vi "Logging Message Loop.vi"(8 "error in (no error)":errorcluster, 10 "Data Queue":refnum<queue>, 11 "Message Queues":T2) -> (0 "error out":errorcluster)   [LabVIEW 2018, in "System Logging.lvlib" / "Logging.lvlib"]
doc: "The message loop subVI to handle messages pertaining to logging data."
uses:
  Logging.lvlib
  Logging Configuration.ctl
  support/Message Queue/Message Queue.lvlib
  Logging State.ctl
  <vilib>/ErrorRing/Error Ring.xnode
  <vilib>/Utility/error.llb/Error Cluster From Error Code.vi
  support/Message Queue/Message Cluster.ctl
  support/Message Queue/All Message Queues.ctl
  Valve Time Stamp.ctl
panel:
  out "Numeric":i32
  out "Boolean 4":bool=TRUE
  out "Boolean 3":bool=TRUE
  out "Boolean 2":bool=TRUE
  out "Trigger times logged":bool=TRUE
  out "Boolean":bool=TRUE
  in  "Cluster 3":T1
  in  "Cluster 2":T1
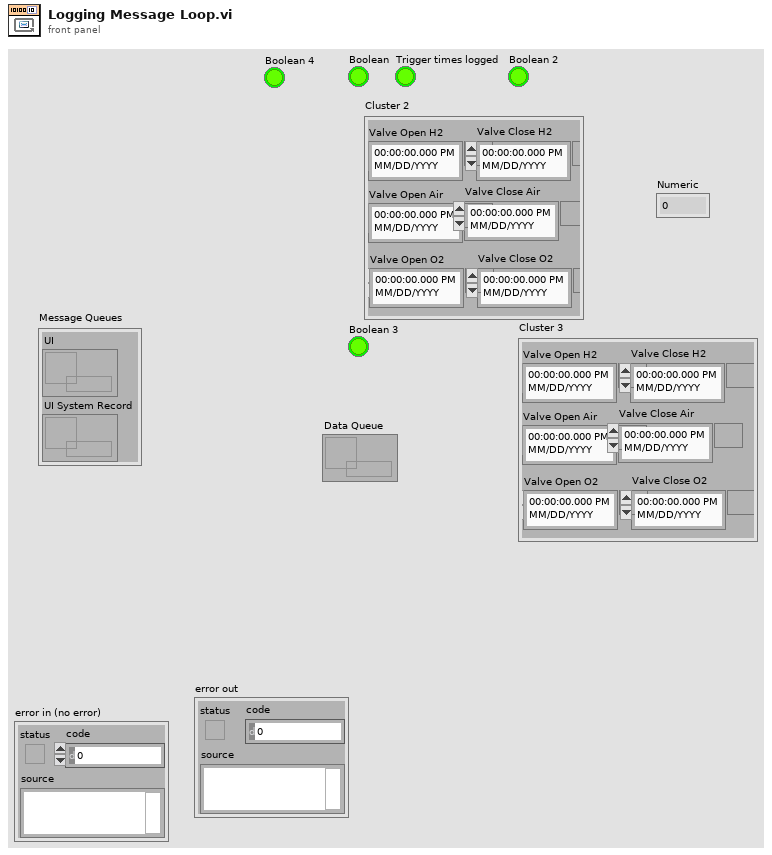
[diagram p1: front panel]
types:
  T1 = typedef "System Logging.lvlib/Valve Time Stamp.ctl" = cluster{"Valve Open Air":timestamp, "Valve Close Air":timestamp, "Valve Open H2":timestamp, "Valve Close H2":timestamp, "Valve Open O2":timestamp, "Valve Close O2":timestamp}
  T2 = typedef "Message Queue.lvlib/All Message Queues.ctl" = cluster{"UI":refnum<queue>, "UI System Record":refnum<queue>}
  T3 = typedef "System Logging.lvlib/Logging.lvlib/Logging State.ctl" = enum16{"Idle", "Logging"}
  T4 = enum16{"open", "open or create", "create or replace", "create", "open (read-only)"}
  T5 = typedef "System Logging.lvlib/Logging.lvlib/Logging Configuration.ctl" = cluster{"Log File Base Path":path, "TDMS File Reference":refnum<k34>, "Log File Base Path 2":path, "TDMS File Reference 2":refnum<k34>}
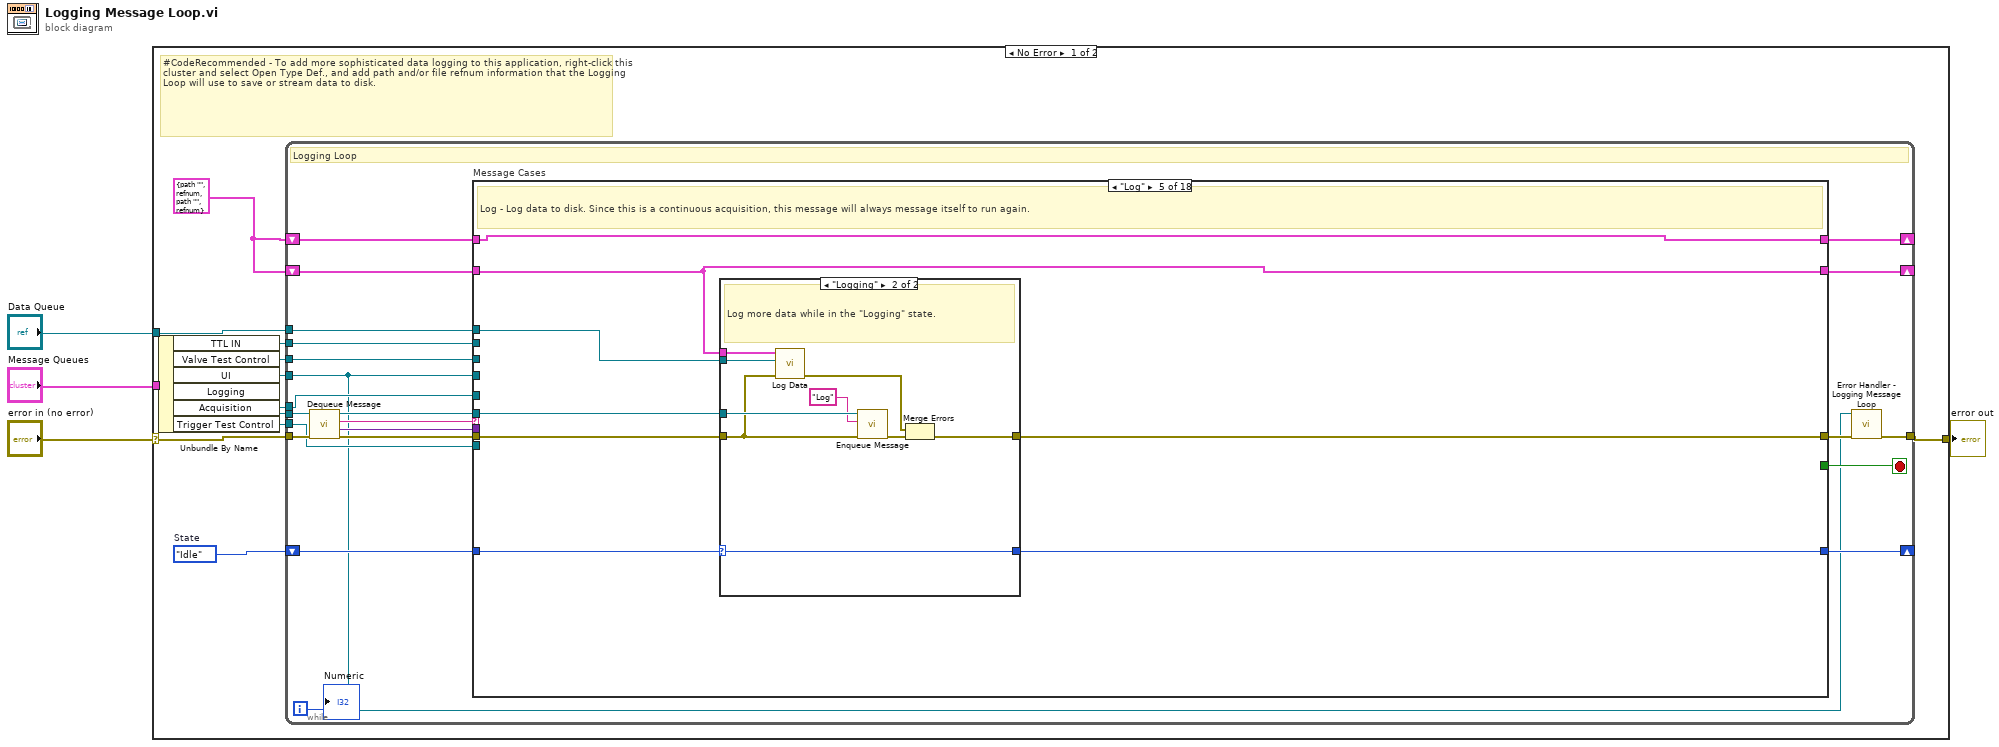
[diagram p0: block diagram]
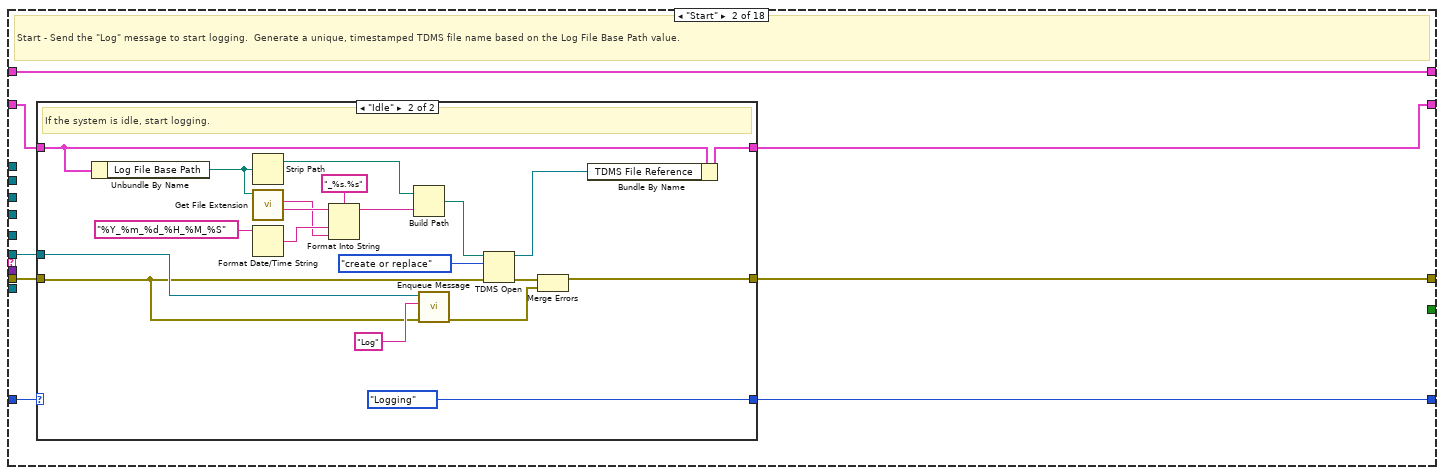
[diagram p3: hidden frame]
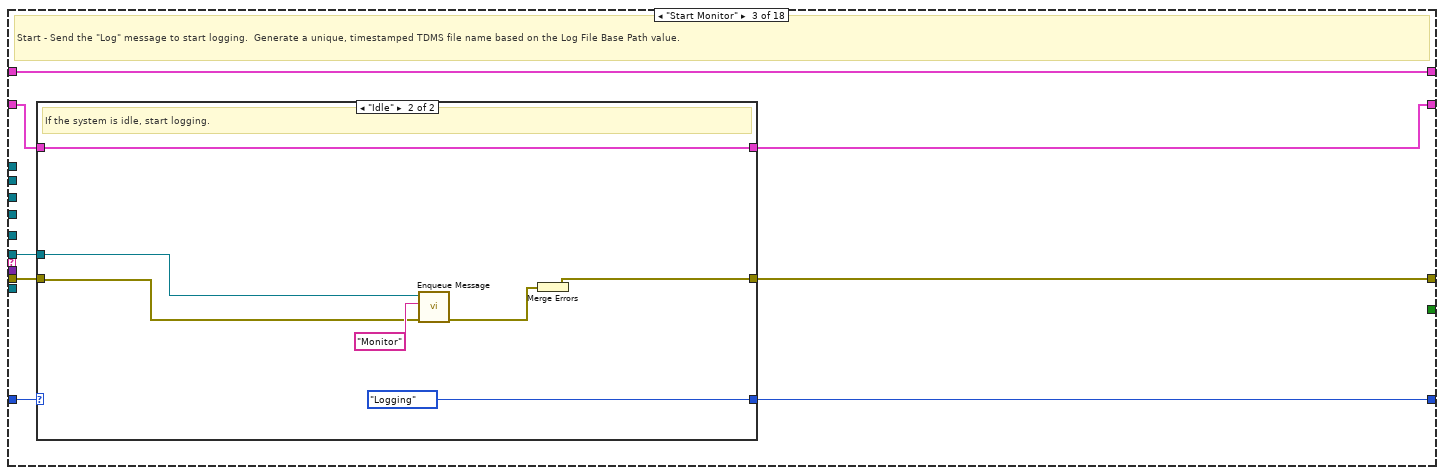
[diagram p5: hidden frame]
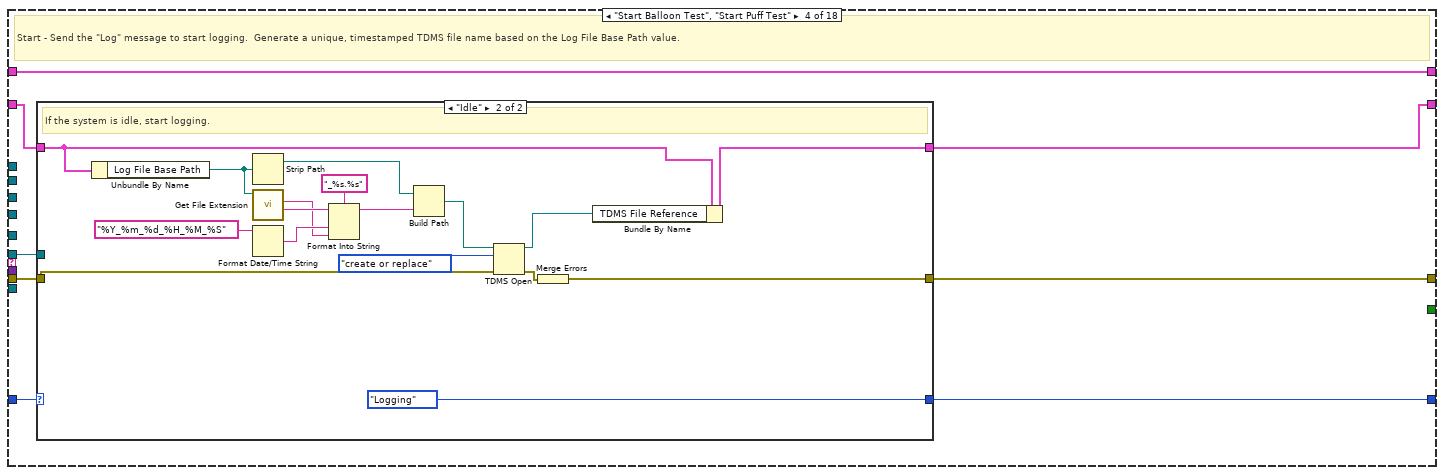
[diagram p7: hidden frame]
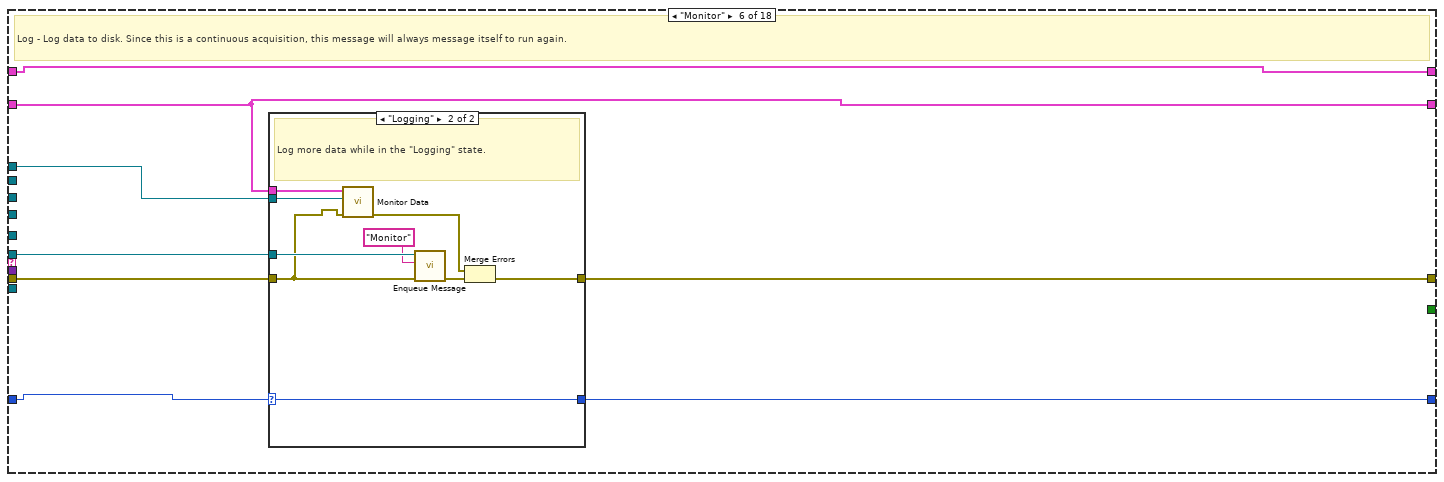
[diagram p10: hidden frame]
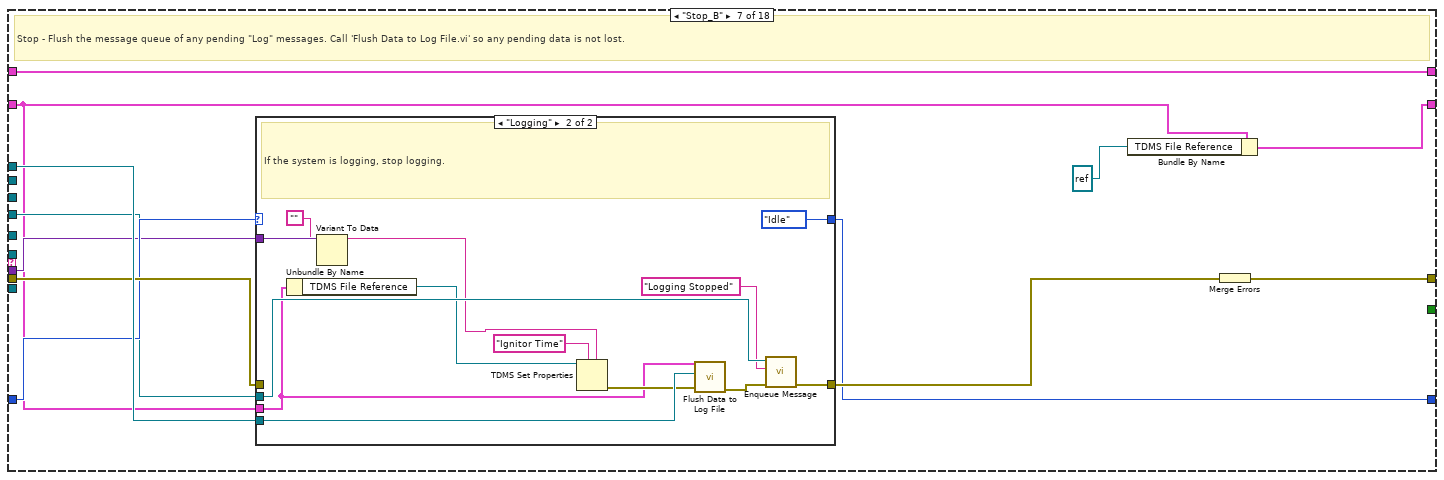
[diagram p12: hidden frame]
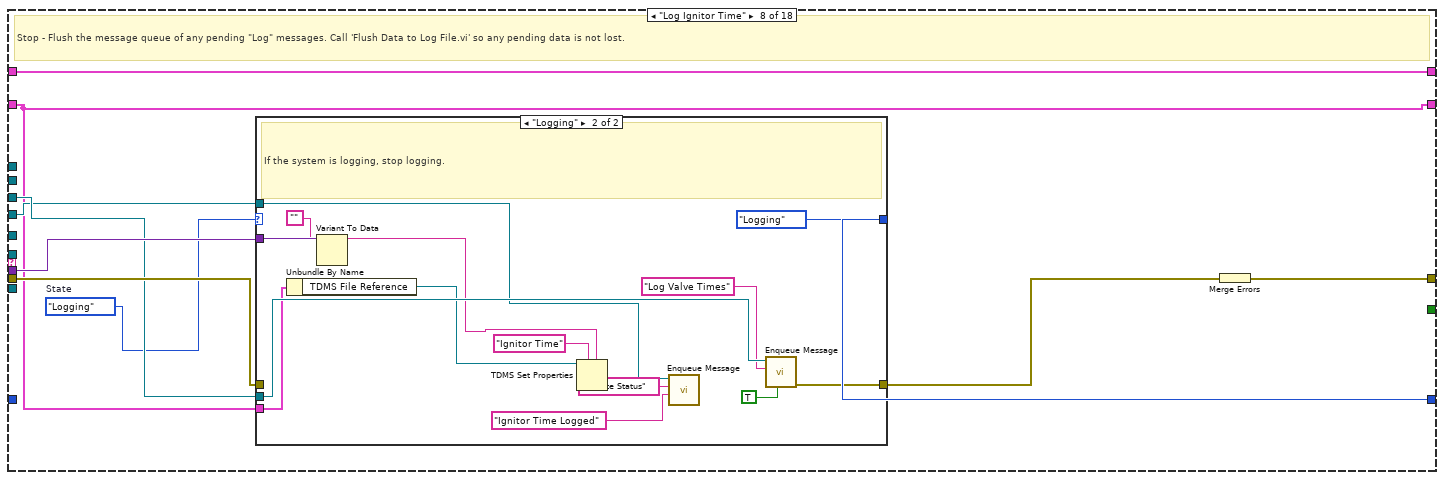
[diagram p14: hidden frame]
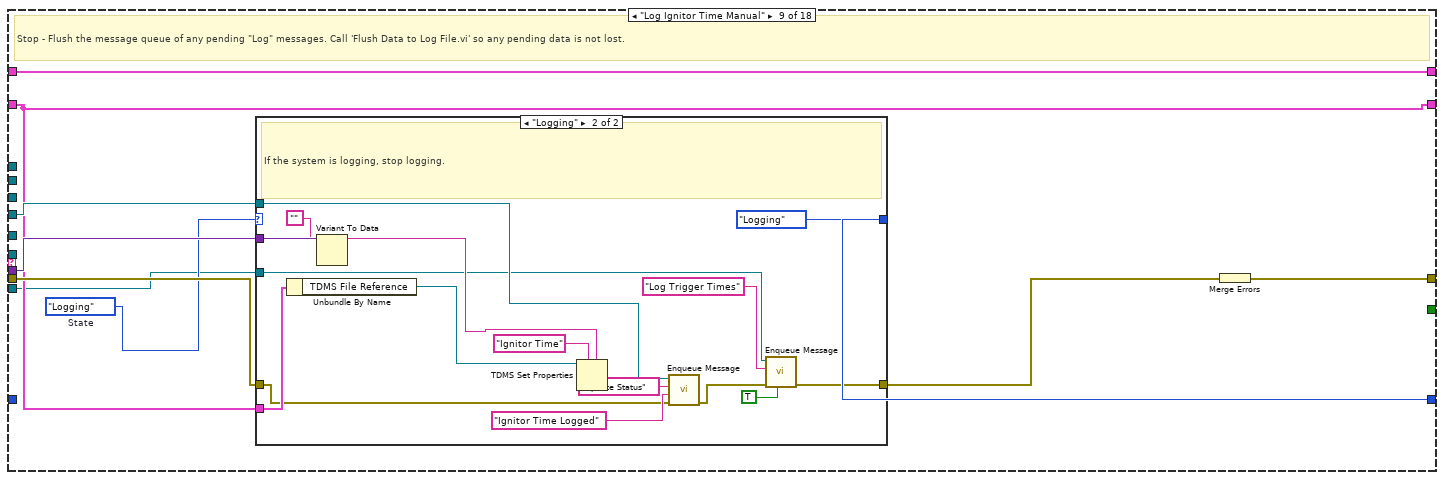
[diagram p16: hidden frame]
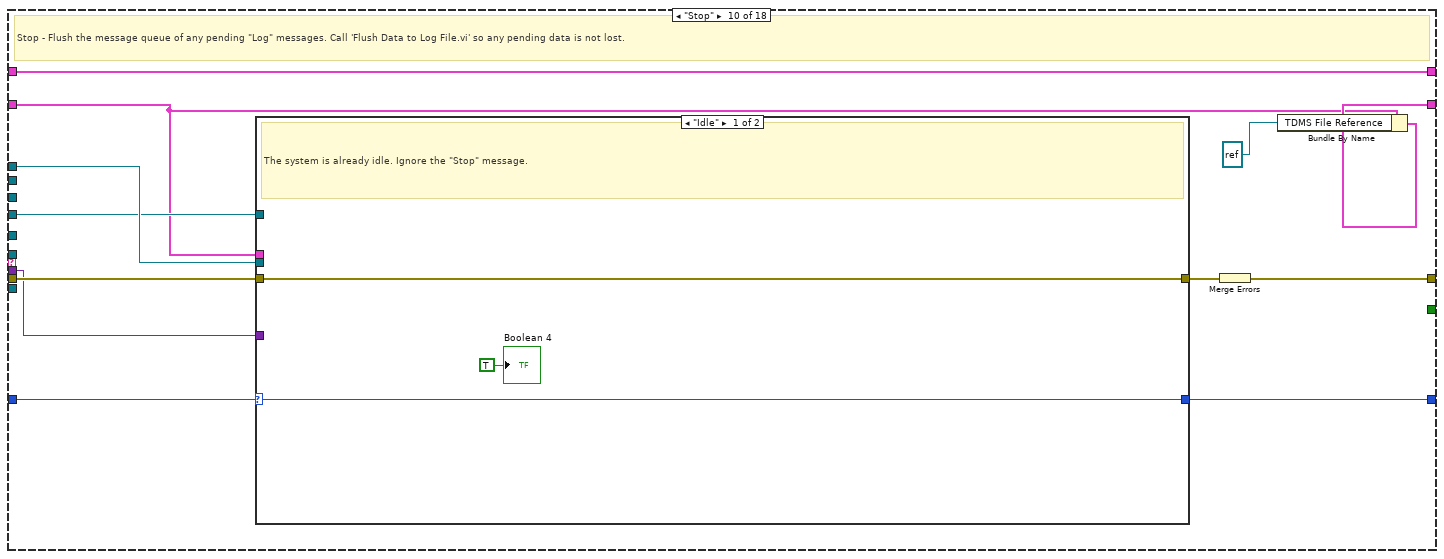
[diagram p18: hidden frame]
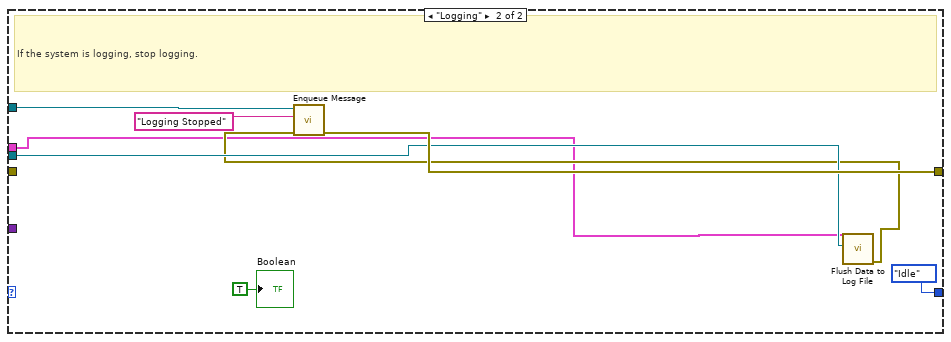
[diagram p19: hidden frame]
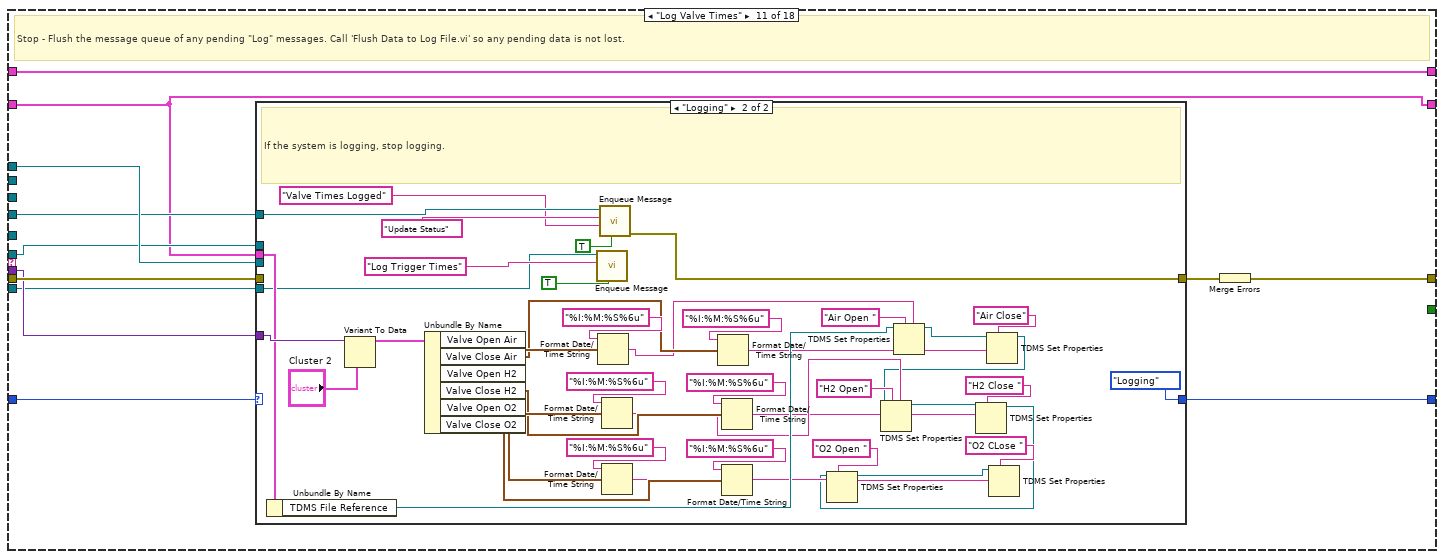
[diagram p20: hidden frame]
diagram:
  n1 = case shown="No Error" "error in (no error)" {
    selector: "error in (no error)" -> [w13 w506]
    tunnel: "Message Queues" -> [w16 _]
    tunnel: [w14 w506] -> w3
    tunnel: "Data Queue" -> [w12 _]
    frame No Error {
      w10 = Logging_State."Idle"  # State
      w7 = T5 {"Log File Base Path"=path "", "TDMS File Reference"=refnum, "Log File Base Path 2"=path "", "TDMS File Reference 2"=refnum} ("Logging Configuration")
      # "#CodeRecommended - To add more sophisticated data logging to this application, right-click this cluster and select Open Type Def., and add path and/or file refnum information that the Logging Loop will use to save or stream data to disk."
      n2 = Unbundle By Name(w16) -> ("TTL IN"=w5:refnum<queue>, "Valve Test Control"=w8:refnum<queue>, "UI"=w11:refnum<queue>, "Logging"=w15:refnum<queue>, "Acquisition"=w9:refnum<queue>, "Trigger Test Control"=w6:refnum<queue>)
      n3 = while {
        tunnel: w15 -> [w25]
        shift-right: [w38] -> _
        shift-left: w7 -> [w23]
        tunnel: w11 -> [w19]
        tunnel: w12 -> [w31]
        shift-right: [w29] -> _
        shift-left: w10 -> [w30]
        tunnel: w13 -> [w36]
        tunnel: [w28] -> w14
        tunnel: w9 -> [w26]
        tunnel: w8 -> [w24]
        shift-right: [w21] -> _
        shift-left: w7 -> [w22]
        tunnel: w6 -> [w20]
        tunnel: w5 -> [w18]
        i -> [w17]
        stop <- w37 stop-if-true
        # "Logging Loop"
        n4 = call "Dequeue Message.vi"("error in (no error)"=w36, "Message Queue"=w25) -> ("error out"=w35:errorcluster, "Message Data"=w33:variant, "Message"=w34:string, "dup Message Queue"=w32:refnum<queue>)  [unwired: 6 in]
        n5 = case "Message Cases" shown="\"Log\"" w34 {
          selector: w34 -> [_ _ _ _ _ _ _ _ _ _ _ _ _ _ _ _ _ w495]
          tunnel: w32 -> [_ w49 w80 w98 w126 w145 _ _ _ _ w265 w322 w383 w427 _ w485 _ _]
          tunnel: w35 -> [w41 w48 w79 w97 w124 w143 w166 w192 w218 w247 w270 w327 w387 w431 w473 w486 w493 _]
          tunnel: [w41 w50 w81 w99 w127 w146 w169 w194 w220 w250 w273 w330 w376 w434 w479 w487 w491 w496] -> w27
          tunnel: w23 -> [w42 w47 w78 w93 w120 w140 w159 w185 w212 w239 w263 w320 w379 w423 w477 w480 w492 w498]
          tunnel: [w42 w46 w77 w96 w120 w140 w158 w185 w212 w240 w263 w320 w379 w423 w474 w480 w492 w498] -> w38
          tunnel: [_ _ _ _ _ _ _ _ _ _ _ _ _ _ _ TRUE _ _] -> w37
          tunnel: w33 -> [_ _ _ _ _ _ w162 w190 w216 w243 w266 w323 w384 w428 w478 _ _ _]
          tunnel: w19 -> [_ _ _ _ _ _ w163 w186 w213 w244 w267 w324 w385 w429 _ _ _ _]
          tunnel: w31 -> [_ _ _ _ w125 w144 w167 _ _ w248 w271 w328 w388 w432 _ w483 _ _]
          tunnel: w30 -> [w40 w45 w76 w95 w123 w139 w165 _ _ w246 w269 w326 _ _ w472 w482 w490 w497]
          tunnel: [w40 w44 w75 w94 w122 w142 w164 w191 w217 w245 w268 w325 w386 w430 w472 w482 w490 w497] -> w29
          tunnel: w26 -> [_ _ _ _ _ _ _ _ _ _ _ _ w381 w425 _ _ _ _]
          tunnel: w24 -> [_ _ _ _ _ _ _ w189 _ _ _ _ _ _ _ _ _ _]
          tunnel: w22 -> [w39 w43 w74 w92 w121 w141 w161 w188 w215 w242 w264 w321 w380 w424 w471 w481 w489 w494]
          tunnel: [w39 w43 w74 w92 w121 w141 w161 w188 w215 w242 w264 w321 w380 w424 w471 w481 w489 w494] -> w21
          tunnel: w20 -> [_ _ _ _ _ _ _ _ w211 _ w262 w319 _ _ _ _ _ _]
          tunnel: w18 -> [_ _ _ _ _ _ _ _ _ _ _ _ w378 _ _ _ _ _]
          frame "Initialize" {
            # "Initialize - gets called when first launched. Currently a no-op."
          }
          frame "Start" {
            # "Start - Send the \"Log\" message to start logging.  Generate a unique, timestamped TDMS file name based on the Log File Base Path value."
            n6 = case shown="\"Idle\"" w45 {
              selector: w45 -> [w52 _]
              tunnel: [w51 w55] -> w50
              tunnel: w49 -> [_ w56]
              tunnel: w48 -> [w51 w54]
              tunnel: w47 -> [w53 w57]
              tunnel: [w53 w59] -> w46
              tunnel: [w52 Logging_State."Logging" ("State")] -> w44
              frame "Logging" {
                # "The system is already logging. Ignore the \"Start\" message."
              }
              frame "Idle" {
                # "If the system is idle, start logging."
                n7 = Unbundle By Name(w57) -> ("Log File Base Path"=w72:path)
                n8 = Strip Path(path=w72) -> (stripped path=w69:path)  [unwired: 1 out]
                n9 = call <vilib>:"Get File Extension.vi"("file"=w72) -> ("filename without extension"=w70:string, "lowercase file extension"=w66:string)  [unwired: 6 in, 3 out]
                n10 = Format Date/Time String(time format string (%c)="%Y_%m_%d_%H_%M_%S") -> (date/time string=w67:string)  [unwired: 2 in]
                n11 = Format Into String(format string="_%s.%s", initial string=w70, w67, w66) -> (resulting string=w65:string)  [unwired: 1 in, 1 out]
                n12 = Build Path(base path=w69, name or relative path=w65) -> (appended path=w64:path)
                n13 = call "Enqueue Message.vi"("error in (no error)"=w54, "Message"="Log", "Message Queue"=w56) -> ("error out"=w62:errorcluster)  [unwired: 7 in, 1 out]
                n14 = TDMS Open(8:w54, 10:T4."create or replace" ("operation (0:open)"), 11:w64) -> (0:w63:errorcluster, 3:w60:refnum<k34>)  [unwired: 4 in]
                n15 = Merge Errors(w63, w62) -> (w55:errorcluster)
                n16 = Bundle By Name(cluster=w57, "TDMS File Reference"=w60) -> (w59:T5)
              }
            }
          }
          frame "Start Monitor" {
            # "Start - Send the \"Log\" message to start logging.  Generate a unique, timestamped TDMS file name based on the Log File Base Path value."
            n17 = case shown="\"Idle\"" w76 {
              selector: w76 -> [w83 _]
              tunnel: [w82 w87] -> w81
              tunnel: w80 -> [_ w88]
              tunnel: w79 -> [w82 w86]
              tunnel: w78 -> [w84 w85]
              tunnel: [w84 w85] -> w77
              tunnel: [w83 Logging_State."Logging" ("State")] -> w75
              frame "Logging" {
                # "The system is already logging. Ignore the \"Start\" message."
              }
              frame "Idle" {
                # "If the system is idle, start logging."
                n18 = call "Enqueue Message.vi"("error in (no error)"=w86, "Message"="Monitor", "Message Queue"=w88) -> ("error out"=w90:errorcluster)  [unwired: 7 in, 1 out]
                n19 = Merge Errors(w90) -> (w87:errorcluster)
              }
            }
          }
          frame "Start Balloon Test", "Start Puff Test" {
            # "Start - Send the \"Log\" message to start logging.  Generate a unique, timestamped TDMS file name based on the Log File Base Path value."
            n20 = case shown="\"Idle\"" w95 {
              selector: w95 -> [w101 _]
              tunnel: [w100 w105] -> w99
              tunnel: w98 -> [_ _]
              tunnel: w97 -> [w100 w104]
              tunnel: w93 -> [w102 w103]
              tunnel: [w102 w107] -> w96
              tunnel: [w101 Logging_State."Logging" ("State")] -> w94
              frame "Logging" {
                # "The system is already logging. Ignore the \"Start\" message."
              }
              frame "Idle" {
                # "If the system is idle, start logging."
                n21 = Unbundle By Name(w103) -> ("Log File Base Path"=w119:path)
                n22 = Strip Path(path=w119) -> (stripped path=w116:path)  [unwired: 1 out]
                n23 = call <vilib>:"Get File Extension.vi"("file"=w119) -> ("filename without extension"=w117:string, "lowercase file extension"=w113:string)  [unwired: 6 in, 3 out]
                n24 = Format Date/Time String(time format string (%c)="%Y_%m_%d_%H_%M_%S") -> (date/time string=w114:string)  [unwired: 2 in]
                n25 = Format Into String(format string="_%s.%s", initial string=w117, w114, w113) -> (resulting string=w112:string)  [unwired: 1 in, 1 out]
                n26 = Build Path(base path=w116, name or relative path=w112) -> (appended path=w111:path)
                n27 = TDMS Open(8:w104, 10:T4."create or replace" ("operation (0:open)"), 11:w111) -> (0:w110:errorcluster, 3:w108:refnum<k34>)  [unwired: 4 in]
                n28 = Merge Errors(w110) -> (w105:errorcluster)
                n29 = Bundle By Name(cluster=w103, "TDMS File Reference"=w108) -> (w107:T5)
              }
            }
          }
          frame "Log" {
            # "Log - Log data to disk. Since this is a continuous acquisition, this message will always message itself to run again."
            n30 = case shown="\"Logging\"" w123 {
              selector: w123 -> [w129 w131]
              tunnel: [w128 w138] -> w127
              tunnel: w126 -> [_ w136]
              tunnel: w125 -> [_ w135]
              tunnel: w124 -> [w128 w130]
              tunnel: w120 -> [_ w132]
              tunnel: [w129 w131] -> w122
              frame "Idle" {
                # "Ignore \"Log\" messages when the logging is idle."
              }
              frame "Logging" {
                # "Log more data while in the \"Logging\" state."
                n31 = call "Log Data.vi"("error in (no error)"=w130, "Data Queue"=w135, "Logging Configuration"=w132) -> ("error out"=w134:errorcluster)  [unwired: 7 in, 1 out]
                n32 = call "Enqueue Message.vi"("error in (no error)"=w130, "Message"="Log", "Message Queue"=w136) -> ("error out"=w137:errorcluster)  [unwired: 7 in, 1 out]
                n33 = Merge Errors(w134, w137) -> (w138:errorcluster)
              }
            }
          }
          frame "Monitor" {
            # "Log - Log data to disk. Since this is a continuous acquisition, this message will always message itself to run again."
            n34 = case shown="\"Logging\"" w139 {
              selector: w139 -> [w148 w153]
              tunnel: [w147 w157] -> w146
              tunnel: w145 -> [_ w155]
              tunnel: w144 -> [_ w150]
              tunnel: w143 -> [w147 w152]
              tunnel: w140 -> [_ w149]
              tunnel: [w148 w153] -> w142
              frame "Idle" {
                # "Ignore \"Log\" messages when the logging is idle."
              }
              frame "Logging" {
                # "Log more data while in the \"Logging\" state."
                n35 = call "Monitor Data.vi"("error in (no error)"=w152, "Data Queue"=w150, "Logging Configuration"=w149) -> ("error out"=w151:errorcluster)  [unwired: 7 in, 1 out]
                n36 = call "Enqueue Message.vi"("error in (no error)"=w152, "Message"="Monitor", "Message Queue"=w155) -> ("error out"=w156:errorcluster)  [unwired: 7 in, 1 out]
                n37 = Merge Errors(w151, w156) -> (w157:errorcluster)
              }
            }
          }
          frame "Stop_B" {
            # "Stop - Flush the message queue of any pending \"Log\" messages. Call 'Flush Data to Log File.vi' so any pending data is not lost."
            n38 = case shown="\"Logging\"" w165 {
              selector: w165 -> [w170 _]
              tunnel: [w171 w183] -> w168
              tunnel: w167 -> [_ w177]
              tunnel: w159 -> [_ w172]
              tunnel: w166 -> [w171 _]
              tunnel: [w170 Logging_State."Idle" ("State")] -> w164
              tunnel: w163 -> [_ w182]
              tunnel: w162 -> [_ w180]
              frame "Idle" {
                # "The system is already idle. Ignore the \"Stop\" message."
              }
              frame "Logging" {
                # "If the system is logging, stop logging."
                n39 = Unbundle By Name(w172) -> ("TDMS File Reference"=w178:refnum<k34>)
                n40 = Variant To Data(type="", Variant=w180) -> (data=w179:string)  [unwired: 1 in, 1 out]
                n41 = TDMS Set Properties(5:w179, 7:"Ignitor Time", 11:w178) -> (0:w173:errorcluster)  [unwired: 3 in, 3 out]
                n42 = call "Flush Data to Log File.vi"("error in (no error)"=w173, "Data Queue"=w177, "Logging Configuration 2"=w172) -> ("error out"=w176:errorcluster)  [unwired: 8 in]
                n43 = call "Enqueue Message.vi"("error in (no error)"=w176, "Message"="Logging Stopped", "Message Queue"=w182) -> ("error out"=w183:errorcluster)  [unwired: 7 in, 1 out]
              }
            }
            n44 = Bundle By Name(cluster=w159, "TDMS File Reference"=refnum<k34> refnum) -> (w158:T5)
            n45 = Merge Errors(w168) -> (w169:errorcluster)
          }
          frame "Log Ignitor Time" {
            w187 = Logging_State."Logging"  # State
            # "Stop - Flush the message queue of any pending \"Log\" messages. Call 'Flush Data to Log File.vi' so any pending data is not lost."
            n46 = case shown="\"Logging\"" w187 {
              selector: w187 -> [w195 _]
              tunnel: [w196 w209] -> w193
              tunnel: w185 -> [_ w203]
              tunnel: w192 -> [w196 _]
              tunnel: [w195 Logging_State."Logging" ("State")] -> w191
              tunnel: w189 -> [_ w208]
              tunnel: w190 -> [_ w206]
              tunnel: w186 -> [_ w200]
              frame "Idle" {
                # "The system is already idle. Ignore the \"Stop\" message."
              }
              frame "Logging" {
                # "If the system is logging, stop logging."
                n47 = Unbundle By Name(w203) -> ("TDMS File Reference"=w204:refnum<k34>)
                n48 = Variant To Data(type="", Variant=w206) -> (data=w205:string)  [unwired: 1 in, 1 out]
                n49 = TDMS Set Properties(5:w205, 7:"Ignitor Time", 11:w204) -> ()  [unwired: 3 in, 4 out]
                n50 = call "Enqueue Message.vi"("Message Data"="Ignitor Time Logged" ("Message"), "Message"="Update Status", "Message Queue"=w200) -> ()  [unwired: 7 in, 2 out]
                n51 = call "Enqueue Message.vi"("Priority Message? (F)"=TRUE, "Message"="Log Valve Times", "Message Queue"=w208) -> ("error out"=w209:errorcluster)  [unwired: 7 in, 1 out]
              }
            }
            n52 = Merge Errors(w193) -> (w194:errorcluster)
          }
          frame "Log Ignitor Time Manual" {
            w214 = Logging_State."Logging"  # State
            # "Stop - Flush the message queue of any pending \"Log\" messages. Call 'Flush Data to Log File.vi' so any pending data is not lost."
            n53 = case shown="\"Logging\"" w214 {
              selector: w214 -> [w221 _]
              tunnel: [w222 w237] -> w219
              tunnel: w212 -> [_ w232]
              tunnel: w218 -> [w222 w224]
              tunnel: [w221 Logging_State."Logging" ("State")] -> w217
              tunnel: w216 -> [_ w235]
              tunnel: w213 -> [_ w229]
              tunnel: w211 -> [_ w225]
              frame "Idle" {
                # "The system is already idle. Ignore the \"Stop\" message."
              }
              frame "Logging" {
                # "If the system is logging, stop logging."
                n54 = Unbundle By Name(w232) -> ("TDMS File Reference"=w233:refnum<k34>)
                n55 = Variant To Data(type="", Variant=w235) -> (data=w234:string)  [unwired: 1 in, 1 out]
                n56 = TDMS Set Properties(5:w234, 7:"Ignitor Time", 11:w233) -> ()  [unwired: 3 in, 4 out]
                n57 = call "Enqueue Message.vi"("error in (no error)"=w224, "Message Data"="Ignitor Time Logged" ("Message"), "Message"="Update Status", "Message Queue"=w229) -> ("error out"=w223:errorcluster)  [unwired: 6 in, 1 out]
                n58 = call "Enqueue Message.vi"("Priority Message? (F)"=TRUE, "error in (no error)"=w223, "Message"="Log Trigger Times", "Message Queue"=w225) -> ("error out"=w237:errorcluster)  [unwired: 6 in, 1 out]
              }
            }
            n59 = Merge Errors(w219) -> (w220:errorcluster)
          }
          frame "Stop" {
            # "Stop - Flush the message queue of any pending \"Log\" messages. Call 'Flush Data to Log File.vi' so any pending data is not lost."
            n60 = case shown="\"Idle\"" w246 {
              selector: w246 -> [w252 _]
              tunnel: [w253 w260] -> w249
              tunnel: w248 -> [_ w257]
              tunnel: w239 -> [_ w255]
              tunnel: w247 -> [w253 _]
              tunnel: [w252 Logging_State."Idle" ("State")] -> w245
              tunnel: w244 -> [_ w259]
              tunnel: w243 -> [_ _]
              frame "Idle" {
                # "The system is already idle. Ignore the \"Stop\" message."
                "Boolean 4" <- TRUE
              }
              frame "Logging" {
                # "If the system is logging, stop logging."
                n61 = call "Flush Data to Log File.vi"("Data Queue"=w257, "Logging Configuration 2"=w255) -> ("error out"=w256:errorcluster)  [unwired: 9 in]
                n62 = call "Enqueue Message.vi"("error in (no error)"=w256, "Message"="Logging Stopped", "Message Queue"=w259) -> ("error out"=w260:errorcluster)  [unwired: 7 in, 1 out]
                "Boolean" <- TRUE
              }
            }
            n63 = Merge Errors(w249) -> (w250:errorcluster)
            n64 = Bundle By Name(cluster=w239, "TDMS File Reference"=refnum<k34> refnum) -> (w240:T5)
          }
          frame "Log Valve Times" {
            # "Stop - Flush the message queue of any pending \"Log\" messages. Call 'Flush Data to Log File.vi' so any pending data is not lost."
            n65 = case shown="\"Logging\"" w269 {
              selector: w269 -> [w274 _]
              tunnel: [w275 w317] -> w272
              tunnel: w271 -> [_ _]
              tunnel: w263 -> [_ w310]
              tunnel: w270 -> [w275 _]
              tunnel: [w274 Logging_State."Logging" ("State")] -> w268
              tunnel: w267 -> [_ w316]
              tunnel: w266 -> [_ w313]
              tunnel: w265 -> [_ _]
              tunnel: w262 -> [_ w277]
              frame "Idle" {
                # "The system is already idle. Ignore the \"Stop\" message."
              }
              frame "Logging" {
                # "If the system is logging, stop logging."
                n66 = Unbundle By Name(w310) -> ("TDMS File Reference"=w311:refnum<k34>)
                n67 = Variant To Data(type="Cluster 2", Variant=w313) -> (data=w312:T1)  [unwired: 1 in, 1 out]
                n68 = Unbundle By Name(w312) -> ("Valve Open Air"=w303:timestamp, "Valve Close Air"=w302:timestamp, "Valve Open H2"=w301:timestamp, "Valve Close H2"=w300:timestamp, "Valve Open O2"=w299:timestamp, "Valve Close O2"=w298:timestamp)
                n69 = call "Enqueue Message.vi"("Priority Message? (F)"=TRUE, "Message"="Log Trigger Times", "Message Queue"=w277) -> ()  [unwired: 7 in, 2 out]
                n70 = Format Date/Time String(time format string (%c)="%I:%M:%S%6u" ("Message"), seconds (now)=w303) -> (date/time string=w291:string)  [unwired: 1 in]
                n71 = call "Enqueue Message.vi"("Priority Message? (F)"=TRUE, "Message Data"="Valve Times Logged", "Message"="Update Status", "Message Queue"=w316) -> ("error out"=w317:errorcluster)  [unwired: 6 in, 1 out]
                n72 = Format Date/Time String(time format string (%c)="%I:%M:%S%6u" ("Message"), seconds (now)=w301) -> (date/time string=w289:string)  [unwired: 1 in]
                n73 = Format Date/Time String(time format string (%c)="%I:%M:%S%6u" ("Message"), seconds (now)=w299) -> (date/time string=w287:string)  [unwired: 1 in]
                n74 = Format Date/Time String(time format string (%c)="%I:%M:%S%6u" ("Message"), seconds (now)=w302) -> (date/time string=w290:string)  [unwired: 1 in]
                n75 = Format Date/Time String(time format string (%c)="%I:%M:%S%6u" ("Message"), seconds (now)=w300) -> (date/time string=w288:string)  [unwired: 1 in]
                n76 = Format Date/Time String(time format string (%c)="%I:%M:%S%6u" ("Message"), seconds (now)=w298) -> (date/time string=w286:string)  [unwired: 1 in]
                n77 = TDMS Set Properties(5:w291, 7:"Air Open ", 11:w311) -> (3:w285:refnum<k34>)  [unwired: 3 in, 3 out]
                n78 = TDMS Set Properties(5:w290, 7:"Air Close", 11:w285) -> (3:w284:refnum<k34>)  [unwired: 3 in, 3 out]
                n79 = TDMS Set Properties(5:w289, 7:"H2 Open", 11:w284) -> (3:w283:refnum<k34>)  [unwired: 3 in, 3 out]
                n80 = TDMS Set Properties(5:w288, 7:"H2 Close ", 11:w283) -> (3:w282:refnum<k34>)  [unwired: 3 in, 3 out]
                n81 = TDMS Set Properties(5:w287, 7:"O2 Open ", 11:w282) -> (3:w281:refnum<k34>)  [unwired: 3 in, 3 out]
                n82 = TDMS Set Properties(5:w286, 7:"O2 CLose ", 11:w281) -> ()  [unwired: 3 in, 4 out]
              }
            }
            n83 = Merge Errors(w272) -> (w273:errorcluster)
          }
          frame "Log Valve Times Balloon" {
            # "Stop - Flush the message queue of any pending \"Log\" messages. Call 'Flush Data to Log File.vi' so any pending data is not lost."
            n84 = case shown="\"Logging\"" w326 {
              selector: w326 -> [w331 _]
              tunnel: [w332 w374] -> w329
              tunnel: w328 -> [_ _]
              tunnel: w320 -> [_ w367]
              tunnel: w327 -> [w332 _]
              tunnel: [w331 Logging_State."Logging" ("State")] -> w325
              tunnel: w324 -> [_ w373]
              tunnel: w323 -> [_ w370]
              tunnel: w322 -> [_ w334]
              tunnel: w319 -> [_ _]
              frame "Idle" {
                # "The system is already idle. Ignore the \"Stop\" message."
              }
              frame "Logging" {
                # "If the system is logging, stop logging."
                n85 = Unbundle By Name(w367) -> ("TDMS File Reference"=w368:refnum<k34>)
                n86 = Variant To Data(type="Cluster 3", Variant=w370) -> (data=w369:T1)  [unwired: 1 in, 1 out]
                n87 = Unbundle By Name(w369) -> ("Valve Open Air"=w360:timestamp, "Valve Close Air"=w359:timestamp, "Valve Open H2"=w358:timestamp, "Valve Close H2"=w357:timestamp, "Valve Open O2"=w356:timestamp, "Valve Close O2"=w355:timestamp)
                n88 = call "Enqueue Message.vi"("Priority Message? (F)"=FALSE, "Message"="Stop", "Message Queue"=w334) -> ()  [unwired: 7 in, 2 out]
                n89 = Format Date/Time String(time format string (%c)="%I:%M:%S%6u" ("Message"), seconds (now)=w360) -> (date/time string=w348:string)  [unwired: 1 in]
                n90 = call "Enqueue Message.vi"("Priority Message? (F)"=TRUE, "Message Data"="Valve Times Logged, Log Complete", "Message"="Update Status End", "Message Queue"=w373) -> ("error out"=w374:errorcluster)  [unwired: 6 in, 1 out]
                n91 = Format Date/Time String(time format string (%c)="%I:%M:%S%6u" ("Message"), seconds (now)=w358) -> (date/time string=w346:string)  [unwired: 1 in]
                n92 = Format Date/Time String(time format string (%c)="%I:%M:%S%6u" ("Message"), seconds (now)=w356) -> (date/time string=w344:string)  [unwired: 1 in]
                n93 = Format Date/Time String(time format string (%c)="%I:%M:%S%6u" ("Message"), seconds (now)=w359) -> (date/time string=w347:string)  [unwired: 1 in]
                n94 = Format Date/Time String(time format string (%c)="%I:%M:%S%6u" ("Message"), seconds (now)=w357) -> (date/time string=w345:string)  [unwired: 1 in]
                n95 = Format Date/Time String(time format string (%c)="%I:%M:%S%6u" ("Message"), seconds (now)=w355) -> (date/time string=w343:string)  [unwired: 1 in]
                n96 = TDMS Set Properties(5:w348, 7:"Air Open ", 11:w368) -> (3:w342:refnum<k34>)  [unwired: 3 in, 3 out]
                n97 = TDMS Set Properties(5:w347, 7:"Air Close", 11:w342) -> (3:w341:refnum<k34>)  [unwired: 3 in, 3 out]
                n98 = TDMS Set Properties(5:w346, 7:"H2 Open", 11:w341) -> (3:w340:refnum<k34>)  [unwired: 3 in, 3 out]
                n99 = TDMS Set Properties(5:w345, 7:"H2 Close ", 11:w340) -> (3:w339:refnum<k34>)  [unwired: 3 in, 3 out]
                n100 = TDMS Set Properties(5:w344, 7:"O2 Open ", 11:w339) -> (3:w338:refnum<k34>)  [unwired: 3 in, 3 out]
                n101 = TDMS Set Properties(5:w343, 7:"O2 CLose ", 11:w338) -> ()  [unwired: 3 in, 4 out]
              }
            }
            n102 = Merge Errors(w329) -> (w330:errorcluster)
          }
          frame "Log Trigger Times" {
            w382 = Logging_State."Logging"  # State
            # "Stop - Flush the message queue of any pending \"Log\" messages. Call 'Flush Data to Log File.vi' so any pending data is not lost."
            n103 = case shown="\"Logging\"" w382 {
              selector: w382 -> [w392 _]
              tunnel: [w393 w403] -> w389
              tunnel: w388 -> [_ _]
              tunnel: w379 -> [_ w419]
              tunnel: w387 -> [w393 w396]
              tunnel: [w392 Logging_State."Logging" ("State")] -> w386
              tunnel: w385 -> [_ w421]
              tunnel: w384 -> [_ w420]
              tunnel: w383 -> [_ _]
              tunnel: w381 -> [_ _]
              tunnel: w378 -> [_ w394]
              frame "Idle" {
                # "The system is already idle. Ignore the \"Stop\" message."
              }
              frame "Logging" {
                # "If the system is logging, stop logging."
                n104 = Unbundle By Name(w419) -> ("TDMS File Reference"=w409:refnum<k34>)
                n105 = Variant To Data(type="", Variant=w420) -> (data=w412:string, error out=w397:errorcluster)  [unwired: 1 in]
                n106 = Merge Errors(w397, w396) -> (w395:errorcluster)
                n107 = String Subset(string=w412, offset (0)=0, length (rest)=14 ("length (rest)")) -> (substring=w410:string)
                n108 = String Subset(string=w412, offset (0)=15, length (rest)=14 ("length (rest)")) -> (substring=w407:string)
                n109 = TDMS Set Properties(5:w410, 7:"Camera Trigger", 8:w395, 11:w409) -> (0:w404:errorcluster, 3:w418:refnum<k34>)  [unwired: 2 in, 2 out]
                n110 = TDMS Set Properties(5:w407, 7:"Spectrum Trigger", 8:w404, 11:w418) -> (0:w401:errorcluster)  [unwired: 2 in, 3 out]
                n111 = call "Enqueue Message.vi"("Priority Message? (F)"=TRUE, "error in (no error)"=w401, "Message"="Log TTL In", "Message Queue"=w394) -> ("error out"=w400:errorcluster)  [unwired: 6 in, 1 out]
                n112 = call "Enqueue Message.vi"("error in (no error)"=w400, "Message Data"="Trigger Times Logged", "Message"="Update Status", "Message Queue"=w421) -> ("error out"=w403:errorcluster)  [unwired: 6 in, 1 out]
                "Trigger times logged" <- TRUE
              }
            }
            n113 = Merge Errors(w389) -> (w377:errorcluster)
            n114 = flat-sequence {
              tunnel: w377 -> [w391]
              tunnel: [w391] -> w376
              frame #0 {
                "Boolean 3" <- TRUE
              }
            }
          }
          frame "Log TTL In" {
            w426 = Logging_State."Logging"  # State
            # "Stop - Flush the message queue of any pending \"Log\" messages. Call 'Flush Data to Log File.vi' so any pending data is not lost."
            n115 = case shown="\"Logging\"" w426 {
              selector: w426 -> [w435 _]
              tunnel: [w436 w452] -> w433
              tunnel: w432 -> [_ _]
              tunnel: w423 -> [_ w467]
              tunnel: w431 -> [w436 w438]
              tunnel: [w435 Logging_State."Logging" ("State")] -> w430
              tunnel: w429 -> [_ w469]
              tunnel: w428 -> [_ w468]
              tunnel: w427 -> [_ w450]
              tunnel: w425 -> [_ _]
              frame "Idle" {
                # "The system is already idle. Ignore the \"Stop\" message."
              }
              frame "Logging" {
                # "If the system is logging, stop logging."
                n116 = Unbundle By Name(w467) -> ("TDMS File Reference"=w458:refnum<k34>)
                n117 = Variant To Data(type="", Variant=w468) -> (data=w441:string, error out=w439:errorcluster)  [unwired: 1 in]
                n118 = Merge Errors(w439, w438) -> (w437:errorcluster)
                n119 = String Subset(string=w441, offset (0)=0, length (rest)=14 ("length (rest)")) -> (substring=w459:string)
                n120 = String Subset(string=w441, offset (0)=15, length (rest)=14 ("length (rest)")) -> (substring=w456:string)
                n121 = TDMS Set Properties(5:w459, 7:"Camera Trigger IN", 8:w437, 11:w458) -> (0:w453:errorcluster, 3:w466:refnum<k34>)  [unwired: 2 in, 2 out]
                n122 = TDMS Set Properties(5:w456, 7:"VIS Spectrum Trigger IN", 8:w453, 11:w466) -> (0:w447:errorcluster, 3:w445:refnum<k34>)  [unwired: 2 in, 2 out]
                n123 = String Subset(string=w441, offset (0)=30, length (rest)=14 ("length (rest)")) -> (substring=w442:string)
                n124 = TDMS Set Properties(5:w442, 7:"IR Spectrum Trigger IN", 8:w447, 11:w445) -> (0:w446:errorcluster)  [unwired: 2 in, 3 out]
                n125 = call "Enqueue Message.vi"("error in (no error)"=w446, "Message"="Stop", "Message Queue"=w450) -> ("error out"=w449:errorcluster)  [unwired: 7 in, 1 out]
                n126 = call "Enqueue Message.vi"("error in (no error)"=w449, "Message Data"="Trigger IN Times Logged, Test Complete", "Message"="Update Status End", "Message Queue"=w469) -> ("error out"=w452:errorcluster)  [unwired: 6 in, 1 out]
                "Boolean 2" <- TRUE
              }
            }
            n127 = Merge Errors(w433) -> (w434:errorcluster)
          }
          frame "Update Settings" {
            # "Update Settings - New settings are available, update the current ones stored in the shift register with the settings sent as part of the message."
            n128 = Variant To Data(error in=w473, type=w477, Variant=w478) -> (data=w476:T5, error out=w475:errorcluster)
            n129 = Select(t=w477, s=w475, f=w476) -> (s? t:f=w474:T5)
            n130 = Merge Errors(w473) -> (w479:errorcluster)
          }
          frame "Exit" {
            # "Don't check the error out. The file reference may have already been released."
            # "Release the Logging queue reference"
            # "Stop the VI"
            # "Exit - Send the Exit message to the UI Message Handler.  Call 'Flush Data to Log File.vi' so any pending data is not lost."
            n131 = Release Queue(queue=w485, error in (no error)=w486) -> (error out=w484:errorcluster)  [unwired: 1 in, 2 out]
            n132 = call "Flush Data to Log File.vi"("Data Queue"=w483, "Logging Configuration 2"=w480) -> ()  [unwired: 9 in, 1 out]
            n133 = Merge Errors(w484) -> (w487:errorcluster)
          }
          frame "---Copy This Frame---" {
            # "Duplicate this frame when creating new messages.  Change this comment in the duplicated frame to describe this message."
            n134 = Merge Errors(w493) -> (w491:errorcluster)
          }
          frame Default {
            # "'Default' case only runs if there is a message that isn't defined in any of the other cases.  Output a programming error."
            n135 = xnode "Error Ring"("parameter 0"=w495) -> ("error out"=w496:errorcluster)
          }
        }
        n136 = call "Error Handler - Logging Message Loop.vi"("error in (no error)"=w27, "Message Queue"=w19) -> ("dup error in"=w28:errorcluster)  [unwired: 8 in, 1 out]
        "Numeric" <- w17
      }
    }
    frame Error {
    }
  }
  "error out" <- w3
